vi "Live Display and capture_1.vi"() -> ()   [LabVIEW 2020]
doc: "The Acquire Every Image (Optimized Performance) example shows the basics of using a ring acquisition. There are some camera restrictions to using this mode that are described in more detail in the block diagram of the VI, but it is recommended to use this method for performance-critical applications when possible."
uses:
  <vilib>/vision/driver/IMAQdx.llb/IMAQdx Acquisition Mode.ctl
  Camera Server/Globals/CamServer global.vi
  <vilib>/vision/driver/NI_Vision_Acquisition_Software.lvlib
  <resource>/objmgr/imaqdx.rc
panel:
  out "Name 1":string
  out "error out":errorcluster
  out "Image count":i32
  out "Image 1":T1(plugin-control)
  in  "Stop":bool
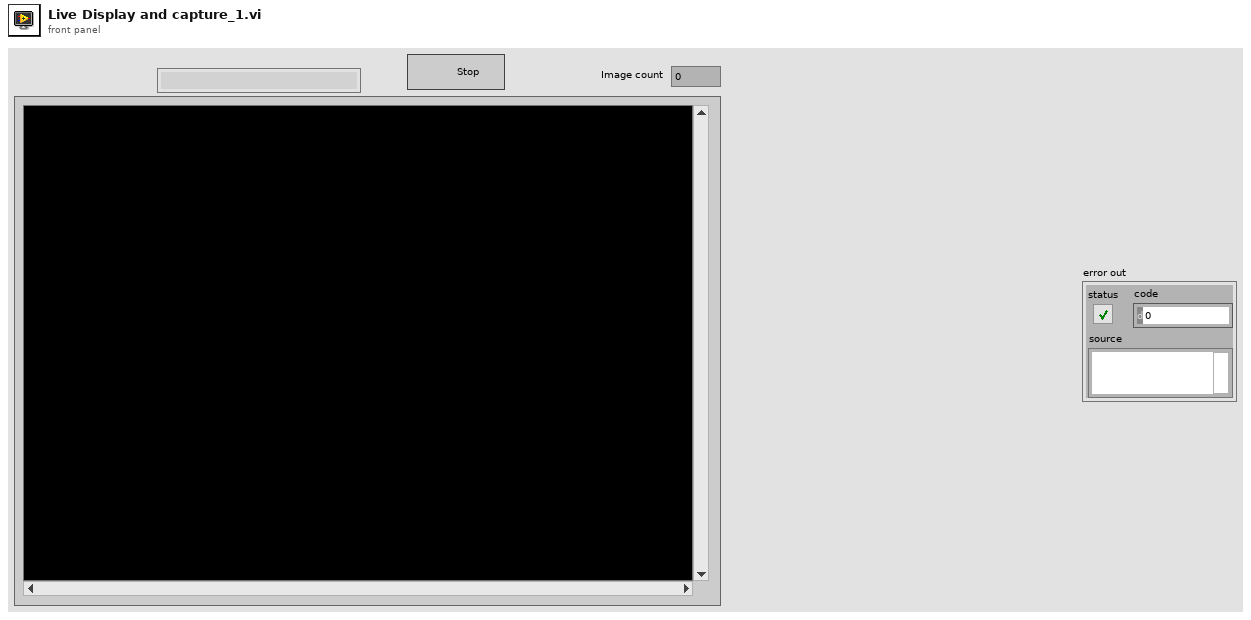
[diagram p1: front panel]
types:
  T1 = typedef "IMAQ Image.ctl" = refnum<image>
  T2 = typedef "NI_Vision_Acquisition_Software.lvlib/IMAQdx Acquisition Mode.ctl" = enum32{"One Shot", "Continuous"}
  T3 = typedef "Camera enum.ctl" = string
  T4 = typedef "IMAQdx.ctl" = refnum<k21>
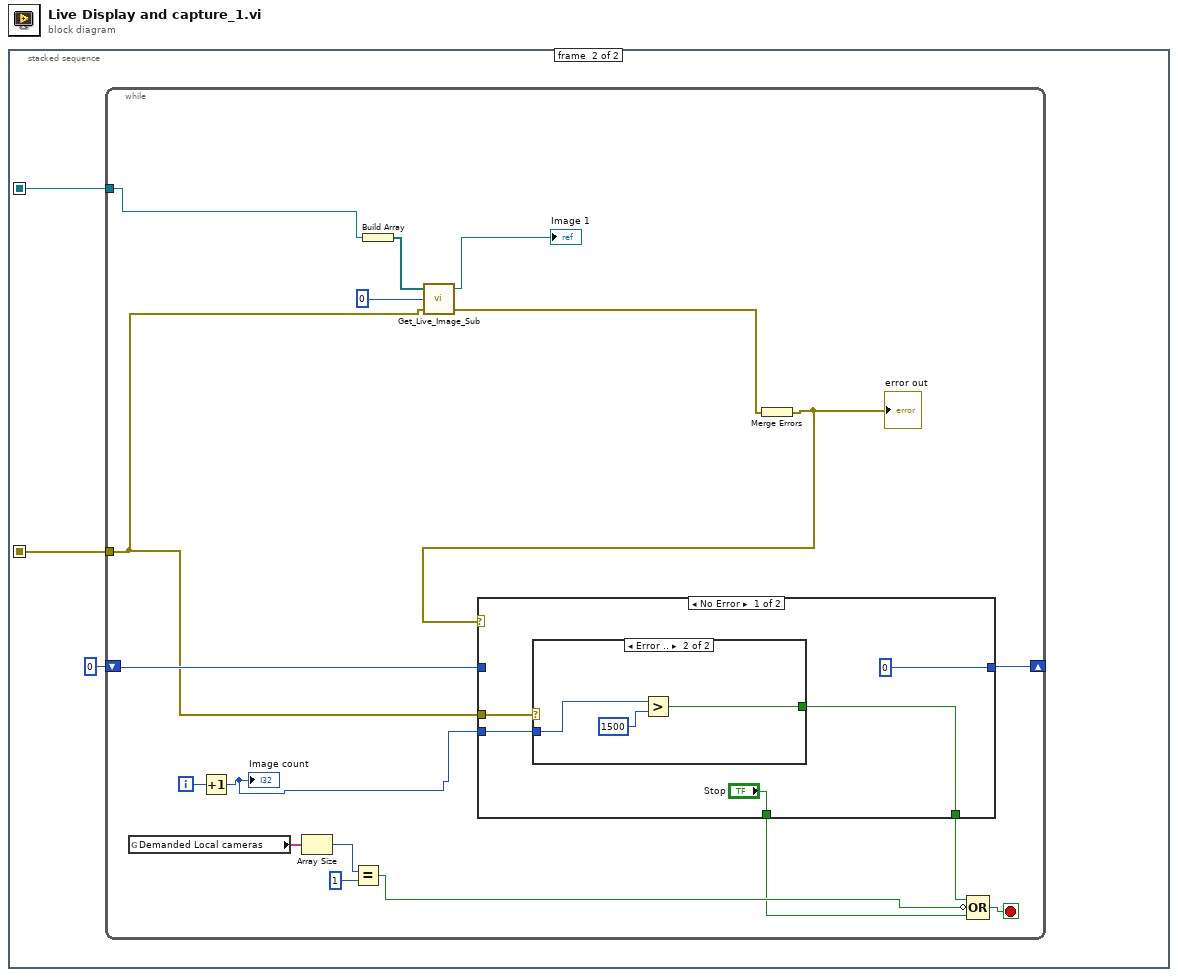
[diagram p0: block diagram]
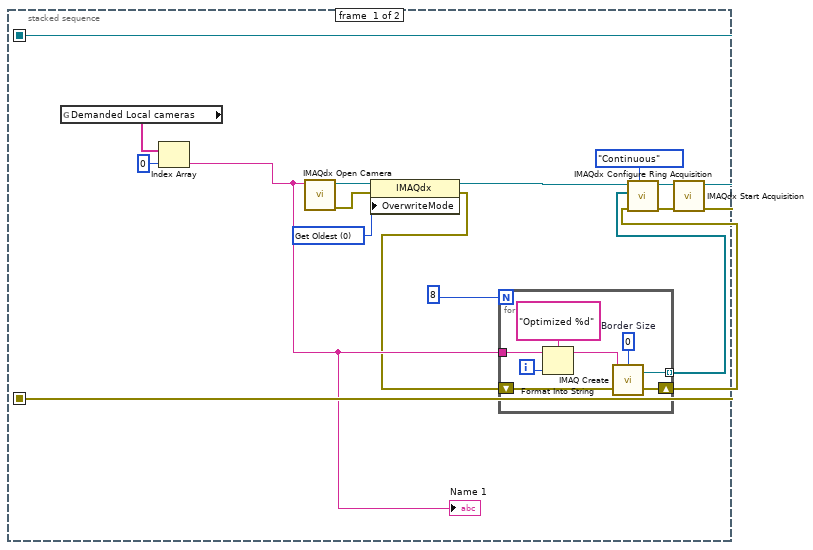
[diagram p2: hidden frame]
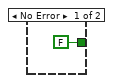
[diagram p3: hidden frame]
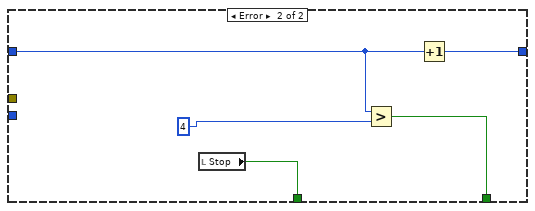
[diagram p4: hidden frame]
diagram:
  n1 = stacked-sequence {
    seq-local: [w16 _] -> [_ w27]
    seq-local: [w15 _] -> [_ w26]
    frame #0 {
      w1 = u32 0 items=["Get Oldest"=0, "Fail"=2, "Get Newest"=3] ("OverwriteMode")
      n2 = global read "CamServer global.vi" "Demanded Local cameras"() -> (w14:T3[])
      n3 = Index Array(array=w14, index=0) -> (element=w12:T3)
      "Name 1" <- w12
      n4 = call <vilib>:"IMAQdx Open Camera.vi"("Session In"=w12) -> ("error out"=w11:errorcluster, "Session Out"=w10:T4)  [unwired: 2 in, 7 out]
      n5 = property class="IMAQdx"(reference=w10, error in=w11, "OverwriteMode"=w1) -> (reference out=w6:T4, error out=w5:errorcluster)
      n6 = for {
        N: 8 ("Number of Images") -> [_]
        tunnel: [w23] -> w3 mode=indexing
        shift-right: [w22] -> w4
        shift-left: w5 -> [w24]
        tunnel: w12 -> [w17]
        i -> [w21]
        w18 = 0  # Border Size
        n7 = Format Into String(format string="Optimized %d" ("Image Name"), initial string=w17, w21) -> (resulting string=w20:string)  [unwired: 1 in, 1 out]
        n8 = call "IMAQ Create"("Border Size"=w18, "Image Name"=w20, "error in (no error)"=w24) -> ("New Image"=w23:T1, "error out"=w22:errorcluster)  [unwired: 1 in, 1 out]
      }
      n9 = call <vilib>:"IMAQdx Configure Ring Acquisition.vi"("Mode"=IMAQdx_Acquisition_Mode."Continuous" ("Continuous?"), "error in"=w4, "Images"=w3, "Session In"=w6) -> ("error out"=w8:errorcluster, "Session Out"=w7:T4)  [unwired: 5 in, 1 out]
      n10 = call <vilib>:"IMAQdx Start Acquisition.vi"("error in"=w8, "Session In"=w7) -> ("error out"=w15:errorcluster, "Session Out"=w16:T4)  [unwired: 8 out]
    }
    frame #1 {
      n11 = while {
        tunnel: w27 -> [w36]
        tunnel: w26 -> [w31]
        shift-right: [w34] -> _
        shift-left: 0 -> [w33]
        i -> [w44]
        stop <- w45 stop-if-true
        n12 = global read "CamServer global.vi" "Demanded Local cameras"() -> (w37:T3[])
        n13 = Increment(x=w44) -> (x+1=w32:i32)
        "Image count" <- w32
        n14 = Array Size(array=w37) -> (size(s)=w43:i32)
        n15 = Equal?(x=w43, y=1) -> (x = y?=w42:bool)
        n16 = Build Array(w36) -> (w35:T4[])
        n17 = call "Get_Live_Image_Sub.vi"("error in"=w31, "index"=0 ("y"), "Session Array"=w35) -> ("error out"=w38:errorcluster, "Image"=→"Image 1":T1)  [unwired: 1 in]
        n18 = Merge Errors(w38) -> (w28:errorcluster)
        "error out" <- w28
        n19 = case shown="No Error" w28 {
          tunnel: [0 w59] -> w34
          tunnel: w33 -> [_ w58]
          tunnel: [w47 w57] -> w29
          tunnel: w31 -> [w49 _]
          tunnel: w32 -> [w48 _]
          tunnel: ["Stop" w55] -> w30
          frame No Error {
            n20 = case shown="Error .." w49 {
              tunnel: w48 -> [_ w53]
              tunnel: [FALSE w52] -> w47
              frame No Error {
              }
              frame Error {
                n21 = Greater?(x=w53, y=1500) -> (0:w52:bool)
              }
            }
          }
          frame Error {
            n22 = local read "Stop"() -> (w55:bool)
            n23 = Greater?(x=w58, y=4) -> (0:w57:bool)
            n24 = Increment(x=w58) -> (x+1=w59:i32)
          }
        }
        n25 = Compound Arithmetic op=OR(w29, invert w42, w30) -> (w45:bool)
      }
    }
  }
